vi "Station jsObject.vi"(6 "Station Instruments (none)":T1[](array[typedef]), 8 "error in (no error)":errorcluster, 9 "Station Record (empty)":T2, 10 "Station jsObject Name (\"\")":string, 11 "Previous String (\"\")":string) -> (0 "error out":errorcluster, 2 "Station jsObject":string, 3 "Station jsObject Definition":string)   [LabVIEW 2011]
uses:
  Station Record.ctl
  Instruments/Instrument Record.ctl
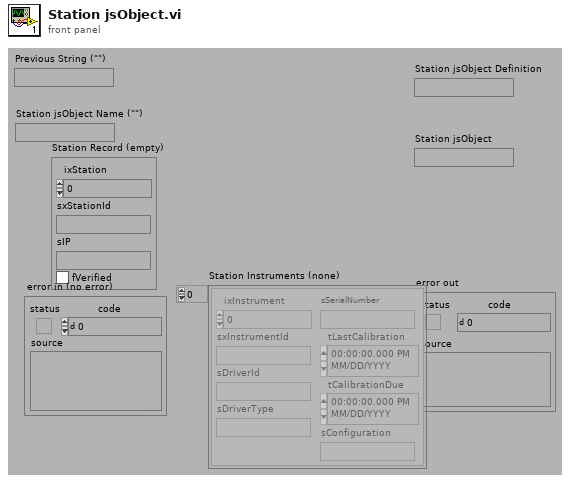
[diagram p1: front panel]
types:
  T1 = typedef "Instrument Record.ctl" = cluster{"ixInstrument":i32, "sxInstrumentId":string, "sDriverId":string, "sDriverType":string, "sSerialNumber":string, "tLastCalibration":timestamp, "tCalibrationDue":timestamp, "sConfiguration":string}
  T2 = typedef "Station Record.ctl" = cluster{"ixStation":i32, "sxStationId":string, "sIP":string, "fVerified":bool}
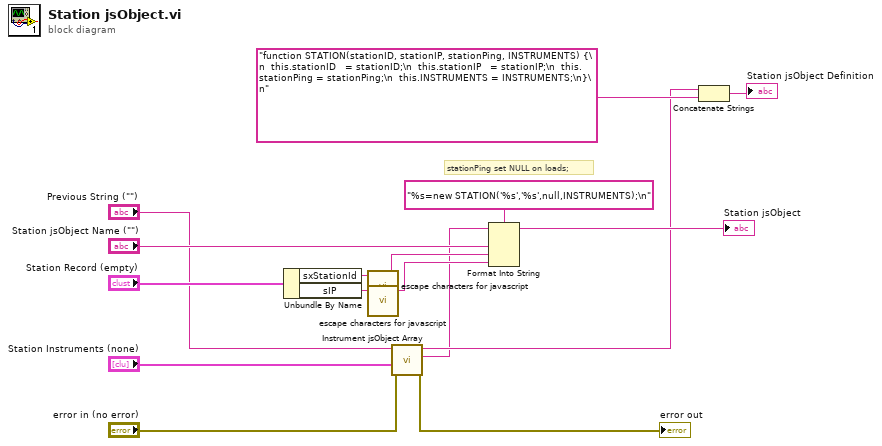
[diagram p0: block diagram]
diagram:
  # "stationPing set NULL on loads;"
  n1 = Unbundle By Name("Station Record (empty)") -> ("sxStationId"=w11:string, "sIP"=w12:string)
  n2 = call "escape characters for javascript.vi"("String (\"\")"=w11) -> ("escaped String"=w10:string)  [unwired: 4 out]
  n3 = call "escape characters for javascript.vi"("String (\"\")"=w12) -> ("escaped String"=w9:string)  [unwired: 4 out]
  n4 = call "Instrument jsObject Array.vi"("error in (no error)"="error in (no error)", "Instruments (empty)"="Station Instruments (none)", "Previous String (\"\")"="Previous String (\"\")") -> ("error out"=→"error out":errorcluster, "Instruments jsObject Array"=w1:string, "Instrument Definition"=w3:string)  [unwired: 1 in, 5 out]
  n5 = Format Into String(format string="%s=new STATION('%s','%s',null,INSTRUMENTS);\n", initial string=w1, "Station jsObject Name (\"\")", w10, w9) -> (resulting string=→"Station jsObject":string)  [unwired: 1 in, 1 out]
  n6 = Concatenate Strings(w3, "function STATION(stationID, stationIP, stationPing, INSTRUMENTS) {\n  this.stationID   = stationID;\n  this.stationIP   = stationIP;\n  this.stationPing = stationPing;\n  this.INSTRUMENTS = INSTRUMENTS;\n}\n") -> (→"Station jsObject Definition":string)
